vi "Set Test Channel Blocks.vi"(8 "error in (no error)":errorcluster, 10 "channel blocks":T1[](array[typedef]) {"buffer offset" format="%d bytes"}, 11 "Mock Transfer in":refnum<class "Mock Transfer.lvclass">) -> (0 "error out":errorcluster, 3 "Mock Transfer out":refnum<class "Mock Transfer.lvclass">)   [LabVIEW 2017, in "Mock Transfer.lvclass"]
uses:
  Mock Transfer.lvclass
  C:/github/data-sharing-framework/Data Sharing Framework Core/Engine/Classes/Transfer/Transfer.lvclass
  Configuration/Public/Controls/DSF Engine Channel Configuration.ctl
  Configuration/Public/Controls/DSF Data Type.ctl
  Engine/Classes/Transfer/Transfer.lvclass/Transfer.ctl
  Engine/Classes/Transfer/Transfer.lvclass
  DSF Core.lvlib
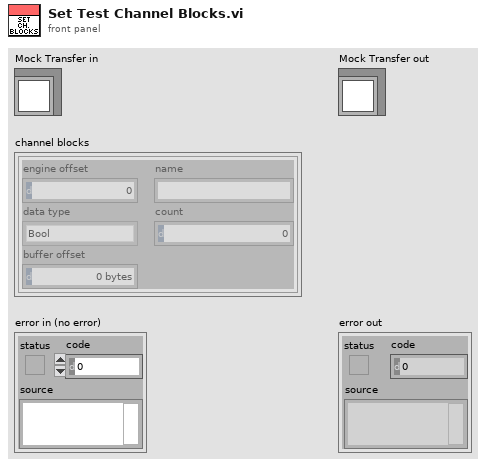
[diagram p1: front panel]
types:
  T1 = typedef "DSF Core.lvlib/DSF Engine Channel Configuration.ctl" = cluster{"engine offset":u64, "name":string, "data type":T2, "count":u64, "buffer offset":u64}
  T2 = typedef "DSF Core.lvlib/DSF Data Type.ctl" = enum8{"Bool", "SGL", "DBL", "I8", "I16", "I32", "I64", "U8", "U16", "U32", "U64"}
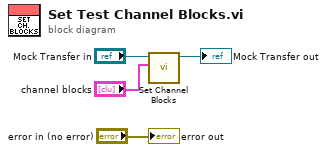
[diagram p0: block diagram]
diagram:
  n1 = call "Set Channel Blocks.vi"("channel blocks"="channel blocks", "Transfer in"="Mock Transfer in") -> ("Transfer out"=→"Mock Transfer out":refnum<class "Mock Transfer.lvclass">)  [unwired: 9 in]
  "error out" <- "error in (no error)"
